vi "Load.vi"   [LabVIEW 2012, in "NI_XML.lvlib"]
doc: "Opens an XML file and allows you to configure the XML parser to validate the file against a schema or Document Type Definition (DTD)."
uses:
  NI_XML.lvlib
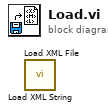
[diagram p0: block diagram]
diagram:
  n1 = call "Load XML String.vi"() -> ()  [unwired: 13 in, 3 out]
  n2 = call "Load XML File.vi"() -> ()  [unwired: 13 in, 3 out]
